vi "createReadCalibrationFrame.vi"(8 "error in (no error)":errorcluster, 9 "TriggerIRQ":bool, 10 "WaitForTrigger":bool, 11 "ILC in":refnum<class "ILC.lvclass">) -> (0 "error out":errorcluster, 2 "TxFrame":T1 {"Data" format="%02x"}, 3 "ILC out":refnum<class "ILC.lvclass">)   [LabVIEW 2016, in "RTILC.lvlib" / "ILC.lvclass"]
uses:
  ILC.lvclass
  Common_RT_Modbus/DataTypes/TxFrame.ctl
  Common_RT_Modbus/DynamicFrameBuilder/DynamicFrameBuilder.lvclass
  ILC.lvclass/ILC.ctl
  Common_RT_Modbus/RTModbus.lvlib
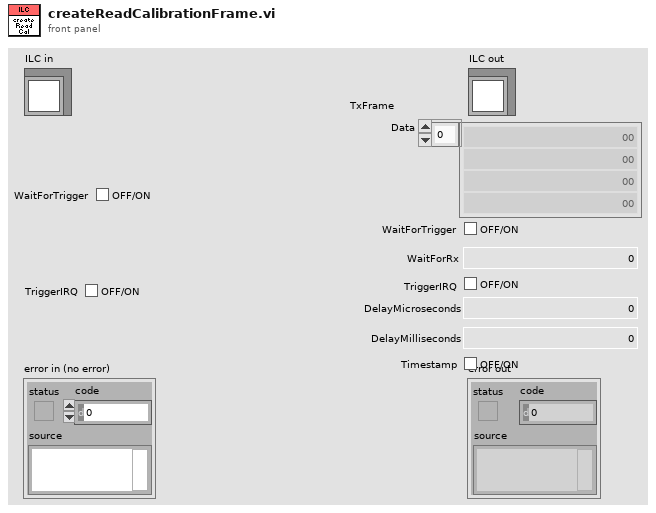
[diagram p1: front panel]
types:
  T1 = typedef "RTModbus.lvlib/TxFrame.ctl" = cluster{"Data":u8[], "WaitForTrigger":bool, "WaitForRx":u16, "TriggerIRQ":bool, "DelayMicroseconds":u16, "DelayMilliseconds":u16, "Timestamp":bool}
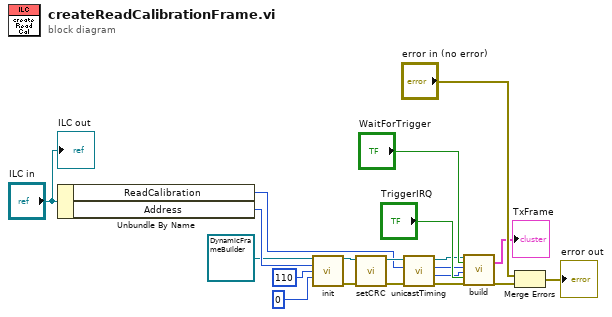
[diagram p0: block diagram]
diagram:
  n1 = Unbundle By Name("ILC in") -> ("ReadCalibration"=w1:u32, "Address"=w16:u8)
  n2 = call "init.vi"("DynamicFrameBuilder in"=refnum<class "DynamicFrameBuilder.lvclass"> refnum ("RTModbus.lvlib:DynamicFrameBuilder.lvclass"), "Address"=w16, "Function"=u8 110, "DataSize"=0) -> ("DynamicFrameBuilder out"=w9:refnum<class "DynamicFrameBuilder.lvclass">, "error out"=w8:errorcluster)  [unwired: 10 in]
  n3 = call "setCRC.vi"("error in (no error)"=w8, "DynamicFrameBuilder in"=w9) -> ("error out"=w2:errorcluster, "DynamicFrameBuilder out"=w7:refnum<class "DynamicFrameBuilder.lvclass">)  [unwired: 8 in]
  n4 = call "unicastTiming.vi"("error in (no error)"=w2, "Latency in"=w1, "DynamicFrameBuilder in"=w7) -> ("error out"=w3:errorcluster, "WaitForRxTimeout"=w4:u16, "Latency out"=w5:u32, "DynamicFrameBuilder out"=w6:refnum<class "DynamicFrameBuilder.lvclass">)  [unwired: 5 in]
  n5 = call "build.vi"("DynamicFrameBuilder in"=w6, "WaitForTrigger"="WaitForTrigger", "Latency"=w5, "WaitForRxTimeout"=w4, "TriggerIRQ"="TriggerIRQ", "error in (no error)"=w3) -> ("TxFrame"=→"TxFrame":T1, "error out"=w11:errorcluster)  [unwired: 11 in, 1 out]
  n6 = Merge Errors("error in (no error)", w11) -> (→"error out":errorcluster)
  "ILC out" <- "ILC in"
